vi "IsClassOrLib.vi"(8 "error in (no error)":errorcluster, 11 "LVFile Name":string) -> (0 "error out":errorcluster, 3 "Is LVClass or Library?":bool)   [LabVIEW 2019, in "Hawkeye.lvlib"]
uses:
  Hawkeye.lvlib
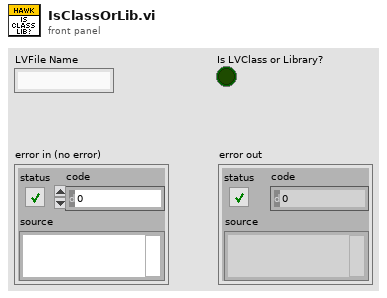
[diagram p1: front panel]
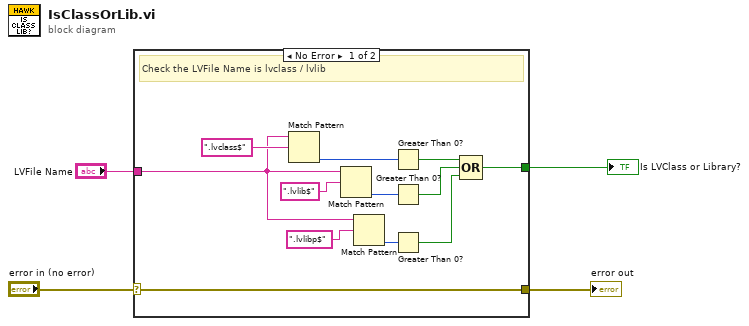
[diagram p0: block diagram]
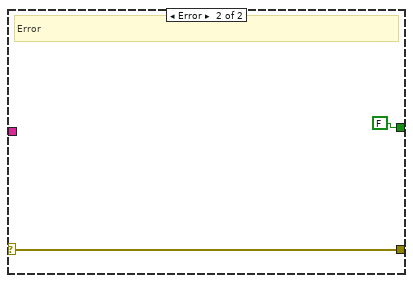
[diagram p2: hidden frame]
diagram:
  n1 = case shown="No Error" "error in (no error)" {
    selector: "error in (no error)" -> [w9 w17]
    tunnel: "LVFile Name" -> [w7 _]
    tunnel: [w10 FALSE] -> w3
    tunnel: [w9 w17] -> w2
    frame No Error {
      # "Check the LVFile Name is lvclass / lvlib"
      n2 = Match Pattern(string=w7, regular expression=".lvclass$" ("pattern")) -> (offset past match=w11:i32)  [unwired: 1 in, 3 out]
      n3 = Match Pattern(string=w7, regular expression=".lvlib$" ("pattern")) -> (offset past match=w12:i32)  [unwired: 1 in, 3 out]
      n4 = Match Pattern(string=w7, regular expression=".lvlibp$" ("pattern")) -> (offset past match=w6:i32)  [unwired: 1 in, 3 out]
      n5 = Greater Than 0?(x=w11) -> (x > 0?=w13:bool)
      n6 = Greater Than 0?(x=w12) -> (x > 0?=w14:bool)
      n7 = Greater Than 0?(x=w6) -> (x > 0?=w5:bool)
      n8 = Compound Arithmetic op=OR(w13, w14, w5) -> (w10:bool)
    }
    frame Error {
      # "Error"
    }
  }
  "Is LVClass or Library?" <- w3
  "error out" <- w2
